vi "Add Call Chain.vi"(8 "error in (no error)":errorcluster, 11 "Logger.Error in":refnum<class "Logger.Error.lvclass">) -> (0 "error out":errorcluster, 3 "Logger.Error out":refnum<class "Logger.Error.lvclass">)   [LabVIEW 2019, in "Logger.Error.lvclass"]
uses:
  Logger.Error.lvclass
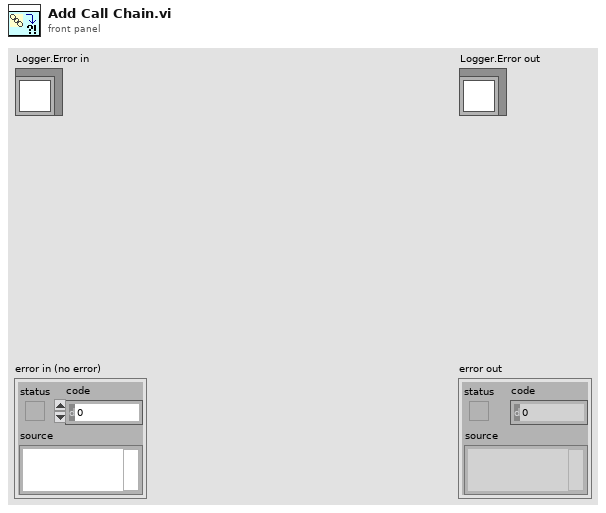
[diagram p1: front panel]
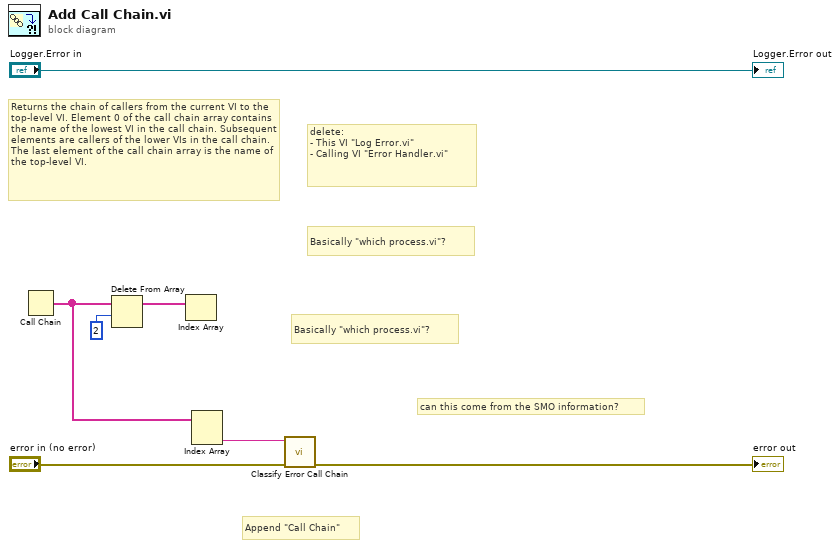
[diagram p0: block diagram]
diagram:
  # "can this come from the SMO information?"
  # "Basically \"which process.vi\"?"
  # "Append \"Call Chain\""
  # "Basically \"which process.vi\"?"
  # "delete:\n- This VI \"Log Error.vi\"\n- Calling VI \"Error Handler.vi\""
  # "Returns the chain of callers from the current VI to the top-level VI. Element 0 of the call chain array contains the name of the lowest VI in the call chain. Subsequent elements are callers of the lower VIs in the call chain. The last element of the call chain array is the name of the top-level VI."
  n1 = Call Chain() -> (call chain=w2:string[])
  n2 = Delete From Array(array=w2, length=2) -> (array with subset deleted=w4:string[])  [unwired: 1 in, 1 out]
  n3 = Index Array(array=w4) -> ()  [unwired: 1 in, 1 out]
  n4 = Index Array(array=w2) -> (element #2=w3:string)  [unwired: 2 in, 1 out]
  n5 = call "Classify Error Call Chain.vi"("Error to Classify"="error in (no error)", "String"=w3) -> ("Classified Error"=→"error out":errorcluster)  [unwired: 9 in]
  "Logger.Error out" <- "Logger.Error in"
